vi "pack_into_wf_array.vi"(9 "name":string, 10 "value":dbl, 11 "time":timestamp) -> (3 "waveform_array":waveform(dbl)[](array[waveform])=[{"t0"=timestamp(0 s since 1904-01-01), "dt"=1.0, "Y"=[]}, {"t0"=timestamp(3732035173.078092 s since 1904-01-01), "dt"=1.0, "Y"=[302.8589782714844], "attributes"=variant("NI_ChannelName"=variant(string "T1"))}])   [LabVIEW 2019]
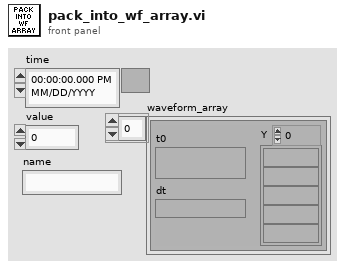
[diagram p1: front panel]
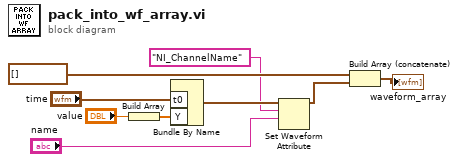
[diagram p0: block diagram]
diagram:
  n1 = Build Array("value") -> (w8:dbl[])
  n2 = Bundle By Name("t0"="time", "Y"=w8) -> (w6:waveform(dbl))  [unwired: 1 in]
  n3 = Set Waveform Attribute(5:"name", 6:"NI_ChannelName" ("name"), 7:w6) -> (3:w7:waveform(dbl))  [unwired: 1 in, 2 out]
  n4 = Build Array (concatenate)(waveform(dbl)[] [], w7) -> (→"waveform_array":waveform(dbl)[])
